vi "msgOutNoClass.vi"(8 "错误输入（无错误）":errorcluster, 10 "字符串":string, 11 "textRef":refnum<vi>) -> (0 "错误输出":errorcluster, 3 "引用输出":refnum<vi>)   [LabVIEW 2011]
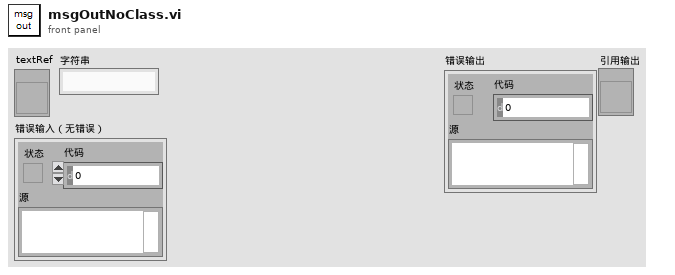
[diagram p1: front panel]
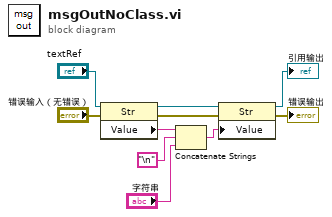
[diagram p0: block diagram]
diagram:
  n1 = property class="Str"(reference="textRef", error in="错误输入（无错误）") -> (reference out=w9:refnum<vi>, error out=w3:errorcluster, "Value"=w8:string)
  n2 = Concatenate Strings(w8, "\n", "字符串") -> (w5:string)
  n3 = property class="Str"(reference=w9, error in=w3, "Value"=w5) -> (reference out=→"引用输出":refnum<vi>, error out=→"错误输出":errorcluster)
